vi "Set Throttles.vi"(8 "error in (no error)":errorcluster, 11 "RDS Helm Actor in":refnum<class "RDS Helm Actor.lvclass">) -> (0 "error out":errorcluster, 3 "RDS Helm Actor out":refnum<class "RDS Helm Actor.lvclass">)   [LabVIEW 2015, in "RDS Helm Actor.lvlib" / "RDS Helm Actor.lvclass"]
uses:
  RDS Helm Actor.lvclass
  Libraries/RDS Child Messages/MCB/MCB Channel.ctl
  Libraries/RDS Framework/RDS Message ID.ctl
  Libraries/RDS Child Messages/MCB/MCB Command Message/MCB Command.lvclass
  RDS Helm Actor.lvclass/RDS Helm Actor.ctl
  Libraries/RDS Framework/RDS Message Class/RDS Message.lvclass/RDS Message.ctl
  Libraries/RDS Child Messages/MCB/MCB Command Message/MCB Command.lvclass/MCB Command.ctl
  Libraries/RDS Framework/RDS Message Class/RDS Message.lvclass
  RDS Parent Actor/RDS Parent Actor/RDS Parent Actor.lvclass
  Libraries/RDS Child Messages/RDS Child Messages.lvlib
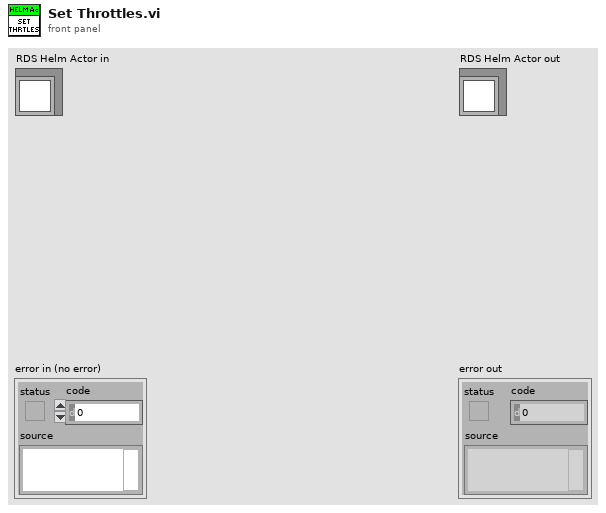
[diagram p1: front panel]
types:
  T1 = typedef "RDS Child Messages.lvlib/MCB Channel.ctl" = enum16{"PORT", "STBD"}
  T2 = typedef "RDS Child Messages.lvlib/RDS Message ID.ctl" = enum16{"RDS Hello World", "String Message", "AIP_Status", "AIP_Command", "GPS_Data", "MCB_Command", "MCB_Status", "Compass_Data", "Depth_Data", "Battery_Data", "Contoller_State", "Set_Mag_Dev", "BTB_Shutdown", "State_Sample_Request", "State_Sample", "PID_Gains_Set", "Helm_Limiter_Set", "Helm_Heading_Command", "Helm_Steering_Command", "Helm_Status", "Controller_Message", "AIP_Set_Min_Depth", "Mission_Controller_State", "Mission_Upload", "Mission_Set_Op_and_Run", "Mission_Settings_Set"}
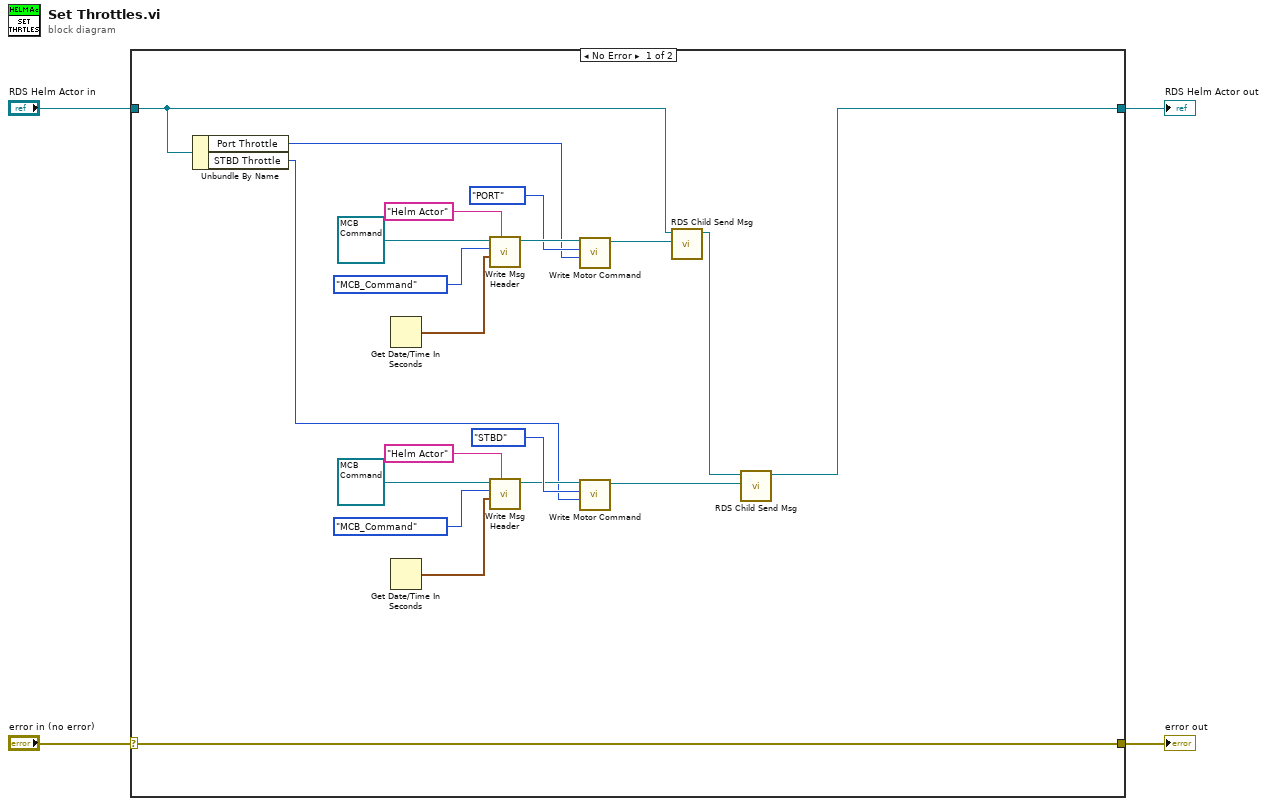
[diagram p0: block diagram]
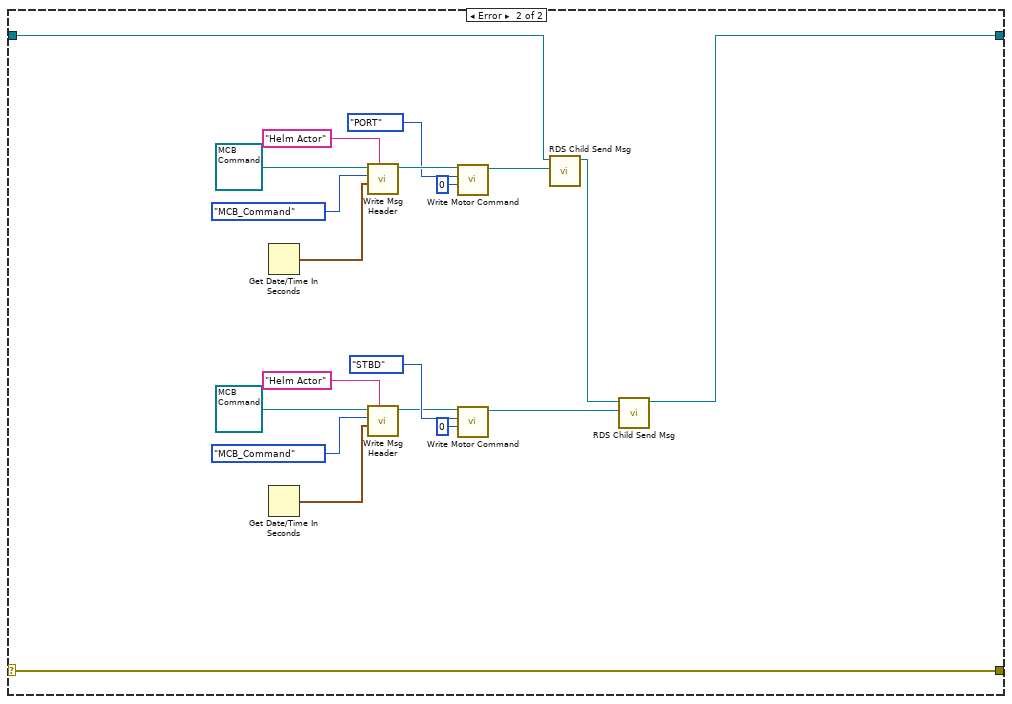
[diagram p2: hidden frame]
diagram:
  n1 = case shown="No Error" "error in (no error)" {
    selector: "error in (no error)" -> [w24 w44]
    tunnel: [w24 w44] -> w3
    tunnel: [w5 w27] -> w1
    tunnel: "RDS Helm Actor in" -> [w6 w28]
    frame No Error {
      n2 = Unbundle By Name(w6) -> ("Port Throttle"=w16:i16, "STBD Throttle"=w8:i16)
      n3 = Get Date/Time In Seconds() -> (seconds since 1Jan1904=w22:timestamp)
      n4 = Get Date/Time In Seconds() -> (seconds since 1Jan1904=w10:timestamp)
      n5 = call "Write Msg Header.vi"("Sender Name"="Helm Actor", "Time Stamp"=w22, "Msg ID"=RDS_Message_ID."MCB_Command", "RDS Message in"=refnum<class "MCB Command.lvclass"> refnum ("RDS Child Messages.lvlib:MCB Command.lvclass")) -> ("RDS Message out"=w19:refnum<class "MCB Command.lvclass">)  [unwired: 6 in, 1 out]
      n6 = call "Write Msg Header.vi"("Sender Name"="Helm Actor", "Time Stamp"=w10, "Msg ID"=RDS_Message_ID."MCB_Command", "RDS Message in"=refnum<class "MCB Command.lvclass"> refnum ("RDS Child Messages.lvlib:MCB Command.lvclass")) -> ("RDS Message out"=w13:refnum<class "MCB Command.lvclass">)  [unwired: 6 in, 1 out]
      n7 = call "Write Motor Command.vi"("Motor Command"=w16, "Motor"=MCB_Channel."PORT", "MCB Command in"=w19) -> ("MCB Command out"=w17:refnum<class "MCB Command.lvclass">)  [unwired: 7 in, 1 out]
      n8 = call "Write Motor Command.vi"("Motor Command"=w8, "Motor"=MCB_Channel."STBD", "MCB Command in"=w13) -> ("MCB Command out"=w15:refnum<class "MCB Command.lvclass">)  [unwired: 7 in, 1 out]
      n9 = call "RDS Child Send Msg.vi"("RDS Message"=w17, "RDS Parent Actor in"=w6) -> ("RDS Parent Actor out"=w7:refnum<class "RDS Helm Actor.lvclass">)  [unwired: 8 in, 1 out]
      n10 = call "RDS Child Send Msg.vi"("RDS Message"=w15, "RDS Parent Actor in"=w7) -> ("RDS Parent Actor out"=w5:refnum<class "RDS Helm Actor.lvclass">)  [unwired: 8 in, 1 out]
    }
    frame Error {
      n11 = Get Date/Time In Seconds() -> (seconds since 1Jan1904=w42:timestamp)
      n12 = Get Date/Time In Seconds() -> (seconds since 1Jan1904=w31:timestamp)
      n13 = call "Write Msg Header.vi"("Sender Name"="Helm Actor", "Time Stamp"=w42, "Msg ID"=RDS_Message_ID."MCB_Command", "RDS Message in"=refnum<class "MCB Command.lvclass"> refnum ("RDS Child Messages.lvlib:MCB Command.lvclass")) -> ("RDS Message out"=w39:refnum<class "MCB Command.lvclass">)  [unwired: 6 in, 1 out]
      n14 = call "Write Msg Header.vi"("Sender Name"="Helm Actor", "Time Stamp"=w31, "Msg ID"=RDS_Message_ID."MCB_Command", "RDS Message in"=refnum<class "MCB Command.lvclass"> refnum ("RDS Child Messages.lvlib:MCB Command.lvclass")) -> ("RDS Message out"=w34:refnum<class "MCB Command.lvclass">)  [unwired: 6 in, 1 out]
      n15 = call "Write Motor Command.vi"("Motor Command"=i16 0, "Motor"=MCB_Channel."PORT", "MCB Command in"=w39) -> ("MCB Command out"=w37:refnum<class "MCB Command.lvclass">)  [unwired: 7 in, 1 out]
      n16 = call "Write Motor Command.vi"("Motor Command"=i16 0, "Motor"=MCB_Channel."STBD", "MCB Command in"=w34) -> ("MCB Command out"=w36:refnum<class "MCB Command.lvclass">)  [unwired: 7 in, 1 out]
      n17 = call "RDS Child Send Msg.vi"("RDS Message"=w37, "RDS Parent Actor in"=w28) -> ("RDS Parent Actor out"=w29:refnum<class "RDS Helm Actor.lvclass">)  [unwired: 8 in, 1 out]
      n18 = call "RDS Child Send Msg.vi"("RDS Message"=w36, "RDS Parent Actor in"=w29) -> ("RDS Parent Actor out"=w27:refnum<class "RDS Helm Actor.lvclass">)  [unwired: 8 in, 1 out]
    }
  }
  "error out" <- w3
  "RDS Helm Actor out" <- w1
